vi "SwissSPAD 1 Load File Info.vi"(8 "error in (no error)":errorcluster, 11 "File Path":path) -> (0 "error out":errorcluster, 1 "Swiss SPAD File Information":T1 {"# Frames" format="%0.0f"; "Scan Increment (step unit)" format="%0.0f"; "Scan Start (step unit)" format="%0.0f"; "# Readouts/Frame" format="%0.0f"; "Initial Micro Shift" format="%0.0f"; "Initial Macro Shift" format="%0.0f"; "# Repetitions" format="%0.0f"; "Pattern Length" format="%0.0f"; "Gate Pattern" format="%064b"; "Recharge Pattern" format="%064b"; "SPAD Off Pattern" format="%064b"}, 2 "size (in bytes)":i64, 3 "Byte Stream File out":refnum<file>)   [LabVIEW 2021, in "SwissSPAD.lvlib"]
uses:
  SwissSPAD1 File Information.ctl
  SwissSPAD.lvlib
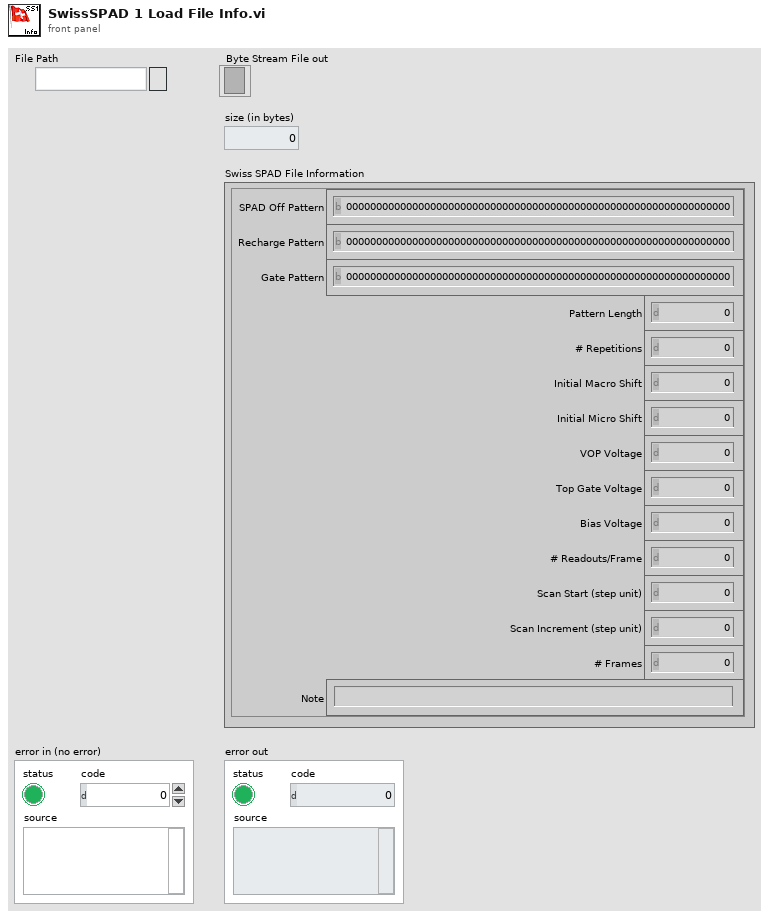
[diagram p1: front panel]
types:
  T1 = typedef "SwissSPAD.lvlib/SwissSPAD1 File Information.ctl" = cluster{"SPAD Off Pattern":u64, "Recharge Pattern":u64, "Gate Pattern":u64, "Pattern Length":u32, "# Repetitions":u32, "Initial Macro Shift":u32, "Initial Micro Shift":u32, "VOP Voltage":dbl, "Top Gate Voltage":dbl, "Bias Voltage":dbl, "# Readouts/Frame":u32, "Scan Start (step unit)":u32, "Scan Increment (step unit)":u32, "# Frames":u32, "Note":string}
  T2 = enum16{"big-endian, network order", "native, host order", "little-endian"}
  T3 = enum16{"open", "replace", "create", "open or create", "replace or create", "replace or create with confirmation"}
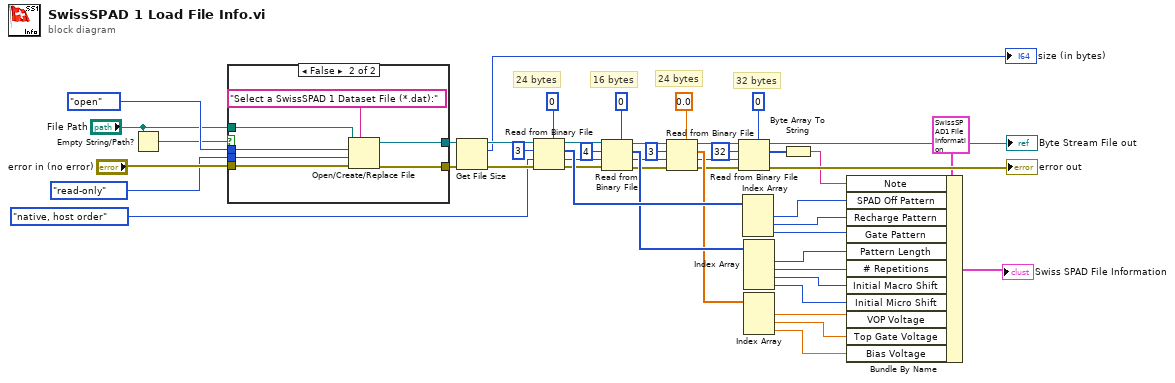
[diagram p0: block diagram]
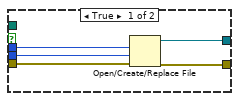
[diagram p2: hidden frame]
diagram:
  w3 = T2."native, host order" ("byte order (0:big-endian, network order)")
  # "32 bytes"
  # "24 bytes"
  # "16 bytes"
  # "24 bytes"
  n1 = Empty String/Path?(string/path="File Path") -> (empty?=w2:bool)
  n2 = case shown="False" w2 {
    tunnel: [w49 w56] -> w27
    tunnel: "error in (no error)" -> [w48 w55]
    tunnel: T3."open" ("operation (0:open)") -> [w47 w54]
    tunnel: enum16{"read/write", "read-only", "write-only"}."read-only" ("access (0:read/write)") -> [w46 w53]
    tunnel: [w45 w52] -> w22
    tunnel: "File Path" -> [_ w51]
    frame True {
      n3 = Open/Create/Replace File(error in=w48, operation (0:open)=w47, access (0:read/write)=w46) -> (refnum out=w45:refnum<file>, error out=w49:errorcluster)  [unwired: 3 in, 1 out]
    }
    frame False {
      n4 = Open/Create/Replace File(file path (use dialog)=w51, error in=w55, prompt="Select a SwissSPAD 1 Dataset File (*.dat):", operation (0:open)=w54, access (0:read/write)=w53) -> (refnum out=w52:refnum<file>, error out=w56:errorcluster)  [unwired: 1 in, 1 out]
    }
  }
  n5 = Get File Size(file=w22, error in=w27) -> (refnum out=w29:refnum<file>, size (in bytes)=→"size (in bytes)":i64, 0:w28:errorcluster)
  n6 = Read from Binary File(5:u64 0 ("U64"), 8:w28, 9:w3, 10:3 ("count (1)"), 11:w29) -> (0:w18:errorcluster, 2:w19:u64[], 3:w17:refnum<file>)  [unwired: 1 in, 1 out]
  n7 = Read from Binary File(5:u32 0 ("U32"), 8:w18, 9:w3, 10:4 ("count (1)"), 11:w17) -> (0:w10:errorcluster, 2:w14:u32[], 3:w11:refnum<file>)  [unwired: 1 in, 1 out]
  n8 = Read from Binary File(5:0.0 ("U32"), 8:w10, 9:w3, 10:3 ("count (1)"), 11:w11) -> (0:w7:errorcluster, 2:w9:dbl[], 3:w8:refnum<file>)  [unwired: 1 in, 1 out]
  n9 = Read from Binary File(5:u8 0 ("U64"), 8:w7, 9:w3, 10:32 ("count (1)"), 11:w8) -> (0:→"error out":errorcluster, 2:w4:u8[], 3:→"Byte Stream File out":refnum<file>)  [unwired: 1 in, 1 out]
  n10 = Index Array(array=w19) -> (element #1=w32:u64, element #2=w33:u64, element #3=w34:u64)  [unwired: 3 in]
  n11 = Index Array(array=w14) -> (element #1=w35:u32, element #2=w36:u32, element #3=w37:u32, element #4=w38:u32)  [unwired: 4 in]
  n12 = Index Array(array=w9) -> (element #1=w39:dbl, element #2=w40:dbl, element #3=w41:dbl)  [unwired: 3 in]
  n13 = Byte Array To String(unsigned byte array=w4) -> (string=w31:string)
  n14 = Bundle By Name(cluster=T1 {"SPAD Off Pattern"=0, "Recharge Pattern"=0, "Gate Pattern"=0, "Pattern Length"=0, "# Repetitions"=0, "Initial Macro Shift"=0, "Initial Micro Shift"=0, "VOP Voltage"=0.0, "Top Gate Voltage"=0.0, "Bias Voltage"=0.0, "# Readouts/Frame"=0, "Scan Start (step unit)"=0, "Scan Increment (step unit)"=0, "# Frames"=0, "Note"=""} ("Swiss SPAD File Information"), "Note"=w31, "SPAD Off Pattern"=w32, "Recharge Pattern"=w33, "Gate Pattern"=w34, "Pattern Length"=w35, "# Repetitions"=w36, "Initial Macro Shift"=w37, "Initial Micro Shift"=w38, "VOP Voltage"=w39, "Top Gate Voltage"=w40, "Bias Voltage"=w41) -> (→"Swiss SPAD File Information":T1)
